vi "Dispense.vi"(8 "error in (no error)":errorcluster, 10 "BallsIn":i32, 11 "object in":refnum<class "HasMoneyState.lvclass">) -> (0 "error out":errorcluster, 2 "BallsOut":i32, 3 "object out":refnum<class "State.lvclass">)   [LabVIEW 2020, in "HasMoneyState.lvclass"]
uses:
  HasMoneyState.lvclass
  C:/Projects/OpenGDS_DesignPatterns/State1/State_class/State.lvclass
  State_class/State.lvclass
  HasMoneyState.lvclass/HasMoneyState.ctl
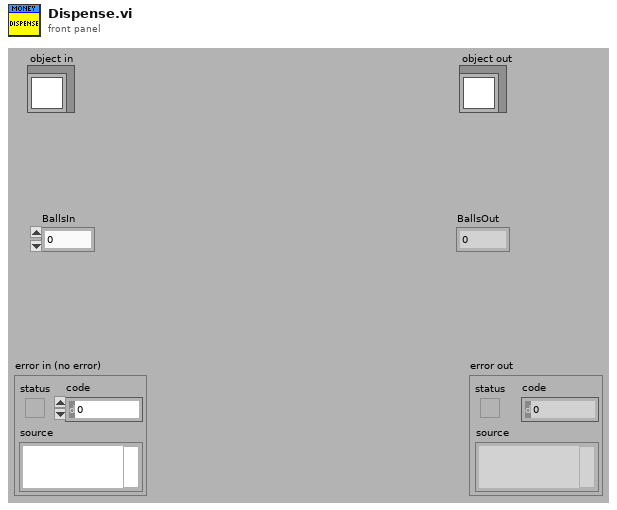
[diagram p1: front panel]
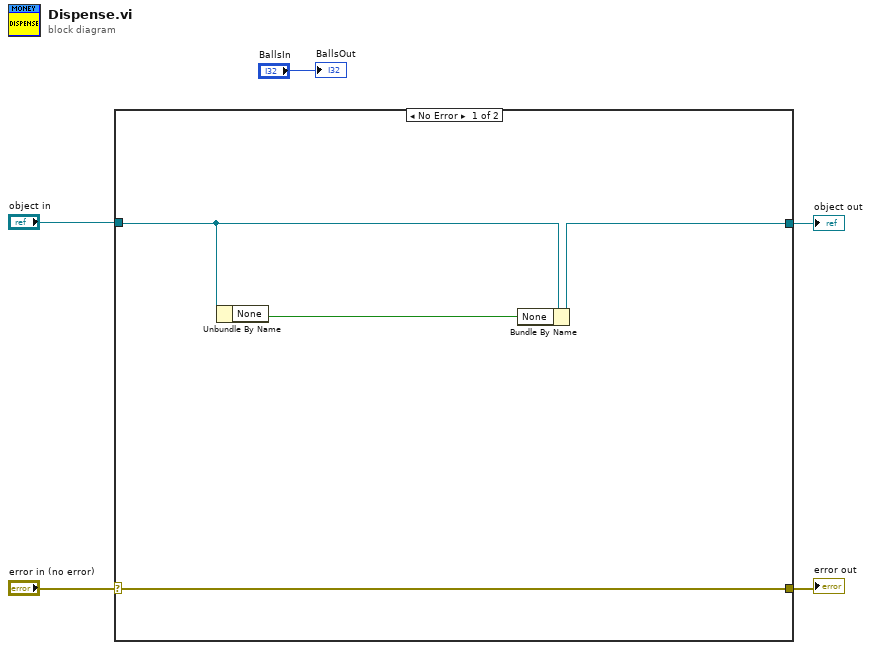
[diagram p0: block diagram]
diagram:
  n1 = case shown="No Error" "error in (no error)" {
    selector: "error in (no error)" -> [w8 w11]
    tunnel: [w8 w11] -> w4
    tunnel: [w6 w10] -> w2
    tunnel: "object in" -> [w7 w10]
    frame No Error {
      n2 = Unbundle By Name(w7) -> ("None"=w9:bool)
      n3 = Bundle By Name(cluster=w7, "None"=w9) -> (w6:refnum<class "HasMoneyState.lvclass">)
    }
    frame Error {
    }
  }
  "error out" <- w4
  "object out" <- w2
  "BallsOut" <- "BallsIn"
